vi "cleanStopped.vi"(7 "input Controls":cluster{"name":string, "type desc":i16[]}[](array[cluster]), 8 "error in (no error)":errorcluster, 11 "vi reference in":refnum<vi>) -> (0 "error out":errorcluster, 2 "stop":bool, 3 "vi reference out":refnum<vi>)   [LabVIEW 2010]
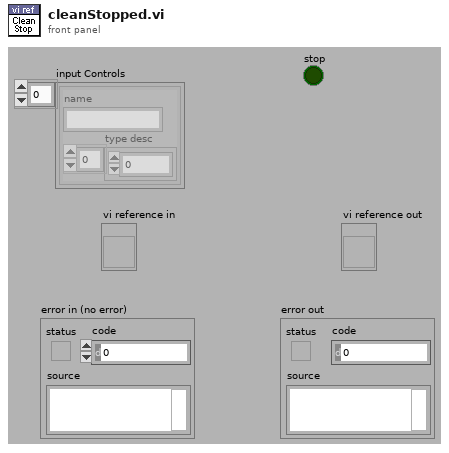
[diagram p1: front panel]
types:
  T1 = enum32{"Bad", "Idle", "Run top level", "Running"}
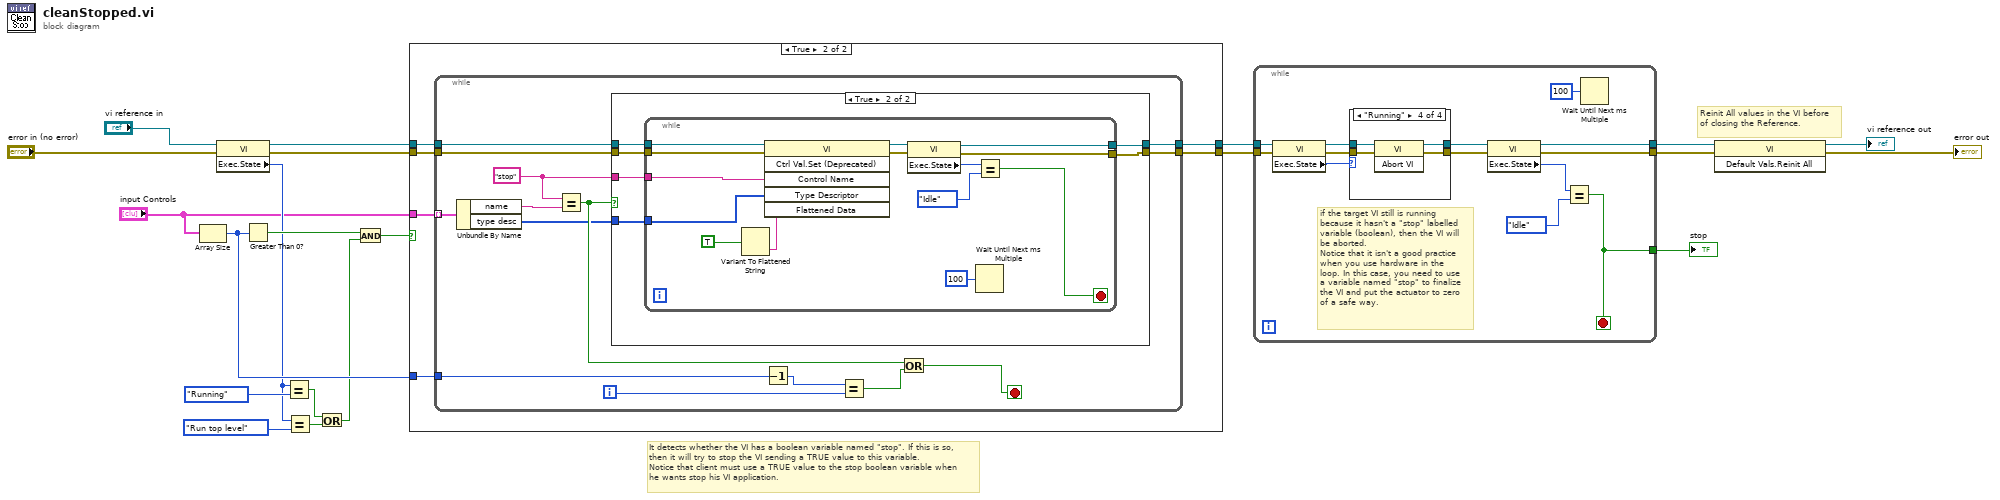
[diagram p0: block diagram]
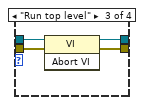
[diagram p4: hidden frame]
diagram:
  # "It detects whether the VI has a boolean variable named \"stop\". If this is so, then it will try to stop the VI sending a TRUE value to this variable.\nNotice that client must use a TRUE value to the stop boolean variable when he wants stop his VI application."
  # "Reinit All values in the VI before of closing the Reference."
  n1 = Array Size(array="input Controls") -> (size(s)=w21:i32)
  n2 = property class="VI"(reference="vi reference in", error in="error in (no error)") -> (reference out=w20:refnum<vi>, error out=w19:errorcluster, "Exec.State"=w14:T1)
  n3 = Greater Than 0?(x=w21) -> (x > 0?=w18:bool)
  n4 = Equal?(x=w14, y=T1."Running") -> (x = y?=w15:bool)
  n5 = Equal?(x=w14, y=T1."Run top level") -> (x = y?=w12:bool)
  n6 = Or(x=w15, y=w12) -> (x .or. y?=w11:bool)
  n7 = And(x=w18, y=w11) -> (x .and. y?=w17:bool)
  n8 = case shown="True" w17 {
    tunnel: "input Controls" -> [_ w29]
    tunnel: w21 -> [_ w28]
    tunnel: w20 -> [w23 w27]
    tunnel: w19 -> [w22 w26]
    tunnel: [w23 w25] -> w5
    tunnel: [w22 w24] -> w4
    frame False {
    }
    frame True {
      n9 = while {
        tunnel: w29 -> [w38] mode=indexing
        tunnel: w28 -> [w41]
        tunnel: w27 -> [w36]
        tunnel: w26 -> [w35]
        tunnel: [w31] -> w25
        tunnel: [w30] -> w24
        i -> [w42]
        stop <- w43 stop-if-true
        w32 = "stop" ("y")
        n10 = Unbundle By Name(w38) -> ("name"=w33:string, "type desc"=w34:i16[])
        n11 = Equal?(x=w32, y=w33) -> (x = y?=w37:bool)
        n12 = case shown="True" w37 {
          tunnel: w36 -> [w45 w51]
          tunnel: w35 -> [w44 w50]
          tunnel: w34 -> [_ w48]
          tunnel: w32 -> [_ w49]
          tunnel: [w45 w47] -> w31
          tunnel: [w44 w46] -> w30
          frame False {
          }
          frame True {
            n13 = while {
              tunnel: w51 -> [w65]
              tunnel: w50 -> [w64]
              tunnel: w49 -> [w60]
              tunnel: w48 -> [w62]
              tunnel: [w54] -> w47
              tunnel: [w53] -> w46
              stop <- w52 stop-if-true
              n14 = Variant To Flattened String(Variant=TRUE) -> (data string=w63:string)  [unwired: 1 out]
              n15 = invoke class="VI" method="Ctrl Val.Set (Deprecated)"(reference=w65, error in=w64, "Control Name"=w60, "Type Descriptor"=w62, "Flattened Data"=w63) -> (reference out=w58:refnum<vi>, error out=w57:errorcluster)  [unwired: 1 in, 4 out]
              n16 = property class="VI"(reference=w58, error in=w57) -> (reference out=w54:refnum<vi>, error out=w53:errorcluster, "Exec.State"=w56:T1)
              n17 = Wait Until Next ms Multiple(millisecond multiple=u32 100) -> ()  [unwired: 1 out]
              n18 = Equal?(x=w56, y=T1."Idle") -> (x = y?=w52:bool)
            }
          }
        }
        n19 = Decrement(x=w41) -> (x-1=w40:i32)
        n20 = Equal?(x=w40, y=w42) -> (x = y?=w39:bool)
        n21 = Or(x=w37, y=w39) -> (x .or. y?=w43:bool)
      }
    }
  }
  n22 = while {
    tunnel: w5 -> [w75]
    tunnel: w4 -> [w74]
    tunnel: [w71] -> w3
    tunnel: [w70] -> w2
    tunnel: [w66] -> w1
    stop <- w66 stop-if-true
    # "if the target VI still is running because it hasn't a \"stop\" labelled variable (boolean), then the VI will be aborted.\nNotice that it isn't a good practice when you use hardware in the loop. In this case, you need to use a variable named \"stop\" to finalize the VI and put the actuator to zero of a safe way."
    n23 = property class="VI"(reference=w75, error in=w74) -> (reference out=w77:refnum<vi>, error out=w76:errorcluster, "Exec.State"=w78:T1)
    n24 = case shown="\"Running\"" w78 {
      tunnel: w77 -> [w80 w82 w86 w90]
      tunnel: w76 -> [w79 w81 w85 w89]
      tunnel: [w80 w82 w83 w88] -> w73
      tunnel: [w79 w81 w84 w87] -> w72
      frame "Bad", Default {
      }
      frame "Idle" {
      }
      frame "Run top level" {
        n25 = invoke class="VI" method="Abort VI"(reference=w86, error in=w85) -> (reference out=w83:refnum<vi>, error out=w84:errorcluster)  [unwired: 1 in, 1 out]
      }
      frame "Running" {
        n26 = invoke class="VI" method="Abort VI"(reference=w90, error in=w89) -> (reference out=w88:refnum<vi>, error out=w87:errorcluster)  [unwired: 1 in, 1 out]
      }
    }
    n27 = property class="VI"(reference=w73, error in=w72) -> (reference out=w71:refnum<vi>, error out=w70:errorcluster, "Exec.State"=w68:T1)
    n28 = Equal?(x=w68, y=T1."Idle") -> (x = y?=w66:bool)
    n29 = Wait Until Next ms Multiple(millisecond multiple=u32 100) -> ()  [unwired: 1 out]
  }
  "stop" <- w1
  n30 = invoke class="VI" method="Default Vals.Reinit All"(reference=w3, error in=w2) -> (reference out=→"vi reference out":refnum<vi>, error out=→"error out":errorcluster)  [unwired: 1 in, 1 out]
